vi "Tosca-Start DI.vi"(0 "Action":enum16{"Stop", "Preview", "Run"}(ring), 7 "Digital Inputs":T1[](array[typedef]), 11 "error in":errorcluster) -> (4 "Task":refnum<k21>, 8 "Bits":i32[](array[numeric]), 15 "error out":errorcluster)   [LabVIEW 2020]
uses:
  Tosca-Digital Input.ctl
  Sub VIs/Tosca-Globals.vi
  epl-vi-lib/Utility VIs/File IO VIs/Configuration File Wrapper VIs/Config-Read Key (string).vi
  <vilib>/DAQmx/create/channels.llb/DAQmx Create Channel (DI-Digital Input).vi
  epl-vi-lib/PXI DAQ VIs/TDT VIs/TDT-Globals.vi
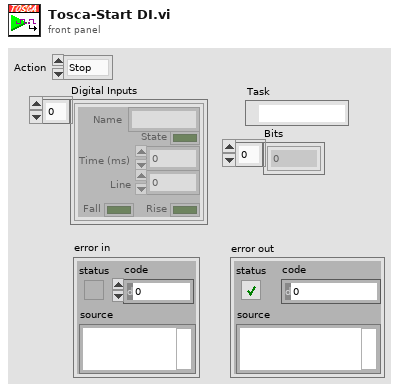
[diagram p1: front panel]
types:
  T1 = typedef "Tosca-Digital Input.ctl" = cluster{"Name":string, "State":bool, "Time (ms)":dbl, "Line":i32, "Rise":bool, "Fall":bool}
  T2 = typedef "TDT-Device Config.ctl" = cluster{"Output":T3, "Input":T5}
  T3 = typedef "TDT-Output source.ctl" = cluster{"Device":T4, "Num":i32}
  T4 = typedef "TDT-Device ID.ctl" = enum16{"None", "PA5", "RP2", "RL2", "RA16", "RV8", "RX5", "RX6", "RX7", "RX8", "RZ2", "RZ5", "RZ6"}
  T5 = typedef "TDT-Input source.ctl" = enum16{"Front Panel", "RA4LI", "RA16LI"}
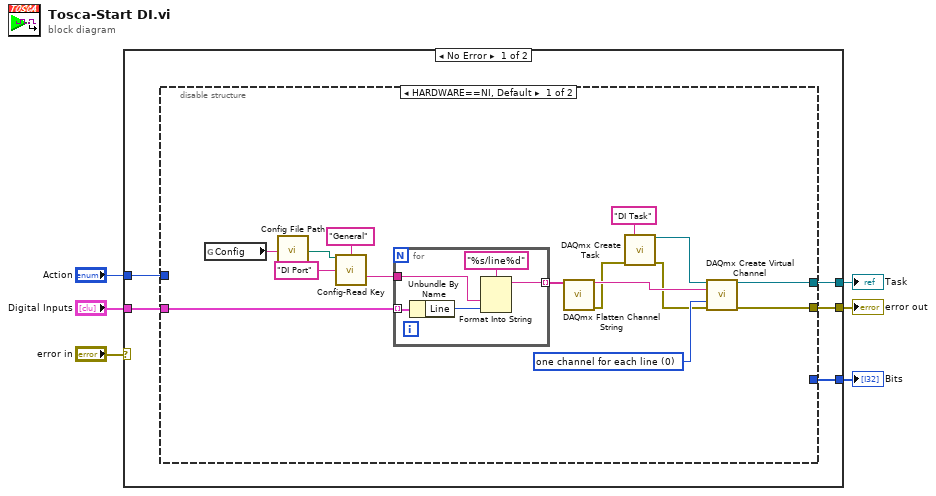
[diagram p0: block diagram]
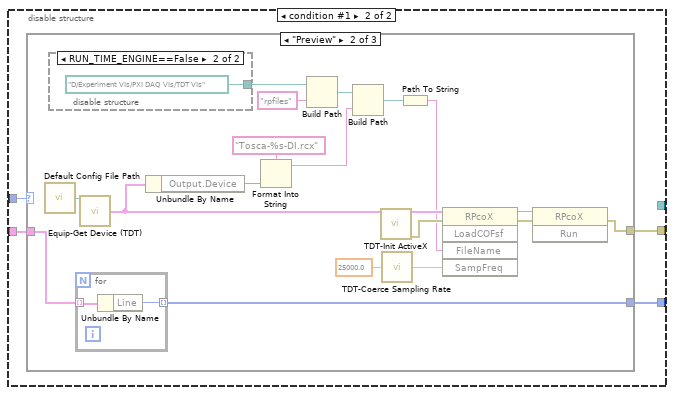
[diagram p2: hidden frame]
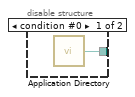
[diagram p4: hidden frame]
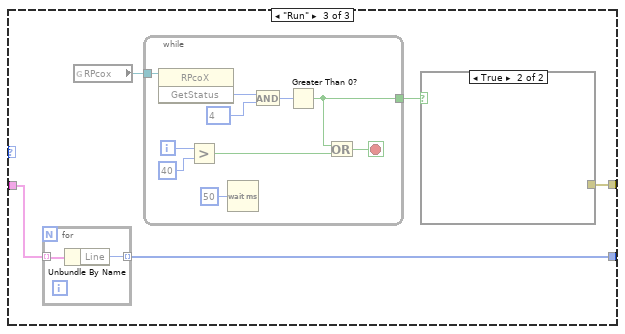
[diagram p5: hidden frame]
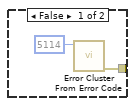
[diagram p6: hidden frame]
diagram:
  n1 = case shown="No Error" "error in" {
    selector: "error in" -> [_ w78]
    tunnel: [w11 w78] -> w6
    tunnel: [w10 _] -> w3
    tunnel: "Digital Inputs" -> [w9 _]
    tunnel: "Action" -> [w8 _]
    tunnel: [w7 _] -> w1
    frame No Error {
      n2 = disable-structure shown="HARDWARE==NI, Default" {
        disable-tunnel: [w26 w35] -> w11
        disable-tunnel: [w21 _] -> w10
        disable-tunnel: w9 -> [w22 w33]
        disable-tunnel: w8 -> [_ w34]
        disable-tunnel: [_ w32] -> w7
        frame condition #0 (active) {
          w25 = 0 items=["one channel for each line", "one channel for all lines"] ("line grouping")
          n3 = global read "Tosca-Globals.vi" "Config"() -> (w14:string)
          n4 = call "Config File Path.vi"("AppName"=w14) -> ("Default config file name"=w17:path)
          n5 = call-poly "Config-Read Key.vi"("configuration file path"=w17, "section"="General", "key"="DI Port") -> ("value"=w18:string)  [unwired: 9 in, 3 out]
          n6 = for {
            tunnel: w22 -> [w31] mode=indexing
            tunnel: [w29] -> w23 mode=indexing
            tunnel: w18 -> [w27]
            n7 = Unbundle By Name(w31) -> ("Line"=w28:i32)
            n8 = Format Into String(format string="%s/line%d", w27, w28) -> (resulting string=w29:string)  [unwired: 2 in, 1 out]
          }
          n9 = call <vilib>:"DAQmx Flatten Channel String.vi"("names in"=w23) -> ("names out"=w24:string, "error out"=w13:errorcluster)  [unwired: 13 in]
          n10 = call <vilib>:"DAQmx Create Task.vi"("new task name"="DI Task" ("name to assign"), "error in"=w13) -> ("task out"=w15:refnum<k21>, "error out"=w12:errorcluster)  [unwired: 12 in]
          n11 = call-poly <vilib>:"DAQmx Create Virtual Channel.vi"("task in"=w15, "lines"=w24, "line grouping"=w25, "error in"=w12) -> ("task out"=w21:refnum<k21>, "error out"=w26:errorcluster)  [unwired: 10 in]
        }
        frame condition #1 {
          n12 = case shown="\"Preview\"" w34 {
            tunnel: [_ w48 w59] -> w35
            tunnel: w33 -> [_ w37 w63]
            tunnel: [_ w36 w62] -> w32
            frame "Stop", Default {
            }
            frame "Preview" {
              n13 = call "Default Config File Path.vi"() -> ("Default config file name"=w47:path)
              n14 = disable-structure shown="RUN_TIME_ENGINE==False" {
                disable-tunnel: [w57 path "D:/Experiment VIs/PXI DAQ VIs/TDT VIs"] -> w44
                frame condition #0 {
                  n15 = call <vilib>:"Application Directory.vi"() -> ("Application Directory"=w57:path)
                }
                frame condition #1 (active) {
                }
              }
              n16 = for {
                tunnel: w37 -> [w56] mode=indexing
                tunnel: [w55] -> w36 mode=indexing
                n17 = Unbundle By Name(w56) -> ("Line"=w55:i32)
              }
              n18 = call "Equip-Get Device (TDT).vi"("Path In"=w47) -> ("TDT-Device Config"=w40:T2)  [unwired: 12 in, 2 out]
              n19 = Unbundle By Name(w40) -> ("Output.Device"=w39:T4)
              n20 = Format Into String(format string="Tosca-%s-DI.rcx", w39) -> (resulting string=w41:string)  [unwired: 2 in, 1 out]
              n21 = Build Path(base path=w44, name or relative path="rpfiles") -> (appended path=w46:path)
              n22 = Build Path(base path=w46, name or relative path=w41) -> (appended path=w43:path)
              n23 = call "TDT-Init ActiveX.vi"("TDT-Device Config"=w40) -> ("TDT-Device Config out"=w54:T2, "error out"=w49:errorcluster)  [unwired: 11 in, 2 out]
              n24 = call "TDT-Coerce Sampling Rate.vi"("Fs (Hz)"=25000.0) -> ("Coerced"=w52:dbl)
              n25 = Path To String(path=w43) -> (string=w38:string)
              n26 = invoke class="RPcoX" method="LoadCOFsf"(reference=w54, error in=w49, "FileName"=w38, "SampFreq"=w52) -> (reference out=w53:refnum<k7>, error out=w50:errorcluster)  [unwired: 1 in, 3 out]
              n27 = invoke class="RPcoX" method="Run"(reference=w53, error in=w50) -> (error out=w48:errorcluster)  [unwired: 1 in, 2 out]
            }
            frame "Run" {
              n28 = for {
                tunnel: w63 -> [w77] mode=indexing
                tunnel: [w76] -> w62 mode=indexing
                n29 = Unbundle By Name(w77) -> ("Line"=w76:i32)
              }
              n30 = global read "TDT-Globals.vi" "RPcox"() -> (w61:refnum<k7>)
              n31 = while {
                tunnel: w61 -> [w75]
                tunnel: [w66] -> w60
                i -> [w70]
                stop <- w67 stop-if-true
                n32 = invoke class="RPcoX" method="GetStatus"(reference=w75) -> ("GetStatus"=w74:i32)  [unwired: 2 in, 2 out]
                n33 = Greater?(x=w70, y=40) -> (0:w68:bool)
                n34 = Wait (ms)(milliseconds to wait=u32 50) -> ()  [unwired: 1 out]
                n35 = And(x=w74, y=4) -> (x .and. y?=w72:i32)
                n36 = Greater Than 0?(x=w72) -> (x > 0?=w66:bool)
                n37 = Or(x=w66, y=w68) -> (x .or. y?=w67:bool)
              }
              n38 = case shown="True" w60 {
                tunnel: [w65 _] -> w59
                frame False {
                  n39 = call <vilib>:"Error Cluster From Error Code.vi"("error code (0)"=5114) -> ("error out"=w65:errorcluster)  [unwired: 8 in]
                }
                frame True {
                }
              }
            }
          }
        }
      }
    }
    frame Error {
    }
  }
  "error out" <- w6
  "Task" <- w3
  "Bits" <- w1
